vi "RGBtoLab.vi"() -> ()   [LabVIEW 8.6]
uses:
  <vilib>/vision/NI_Vision_Development_Module.lvlib
  <vilib>/vision/Image Controls.llb/IMAQ Image.ctl
panel:
  in  "File Path":path
  out "L out":T1
  out "a out":T1
  out "b out":T1
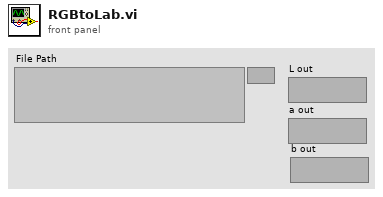
[diagram p1: front panel]
types:
  T1 = typedef "IMAQ Image.ctl" = refnum<image>
  T2 = typedef "Image Type" = u32
  T3 = cluster{"Red (or Hue) value":u8, "Green (or Sat) value":u8, "Blue (or Light or Val) value":u8}[][]
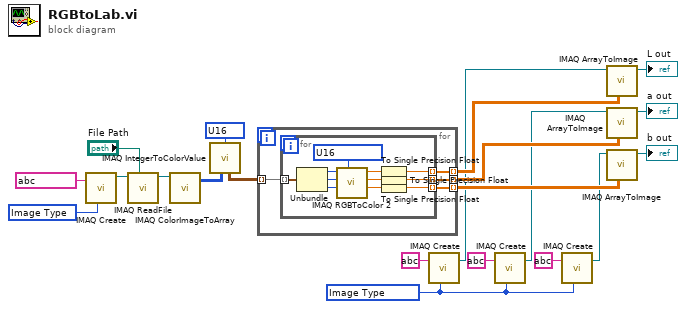
[diagram p0: block diagram]
diagram:
  w15 = T2 ? items=["Grayscale (U8)", "Grayscale (I16)", "Grayscale (SGL)", "Complex (CSG)", "RGB (U32)", "HSL (U32)", "RGB (U64)", "Grayscale (U16)"] ("Image Type")
  w3 = u16 ? items=["RGB", "HSL", "HSV", "HSI"] ("Color Mode")
  w1 = T2 ? items=["Grayscale (U8)", "Grayscale (I16)", "Grayscale (SGL)", "Complex (CSG)", "RGB (U32)", "HSL (U32)", "RGB (U64)", "Grayscale (U16)"] ("Image Type")
  n1 = call "IMAQ Create"("Image Name"=string ?, "Image Type"=w1) -> ("New Image"=w6:T1)  [unwired: 3 in, 1 out]
  n2 = call "IMAQ ReadFile"("File Path"="File Path", "Image"=w6) -> ("Image Out"=w7:T1)  [unwired: 5 in, 4 out]
  n3 = call "IMAQ ColorImageToArray"("Image"=w7) -> ("Image Pixels (U32)"=w2:u32[][])  [unwired: 2 in, 3 out]
  n4 = call "IMAQ IntegerToColorValue"("2D U32 array"=w2, "Color Mode"=w3) -> ("2D Color value array"=w4:T3)  [unwired: 3 in, 3 out]
  n5 = for {
    tunnel: w4 -> [w25] mode=indexing
    tunnel: [w24] -> w16 mode=indexing
    tunnel: [w23] -> w17 mode=indexing
    tunnel: [w22] -> w18 mode=indexing
    n6 = for {
      tunnel: w25 -> [w36] mode=indexing
      tunnel: [w32] -> w24 mode=indexing
      tunnel: [w28] -> w23 mode=indexing
      tunnel: [w27] -> w22 mode=indexing
      w26 = u16 ? items=["RGB", "HSL", "HSV", "HSI", "CIE L*a*b*", "CIE XYZ"] ("Color Mode")
      n7 = Unbundle(w36) -> ("Red (or Hue) value"=w35:u8, "Green (or Sat) value"=w34:u8, "Blue (or Light or Val) value"=w33:u8)
      n8 = call "IMAQ RGBToColor 2"("Color Mode"=w26, "Blue value"=w33, "Green value"=w34, "Red value"=w35) -> ("Blue or Luma or Val or Inten or Z or b*value"=w29:dbl, "Green or Sat or Y or a* value"=w30:dbl, "Red or Hue or X or L* value"=w31:dbl)  [unwired: 3 in, 2 out]
      n9 = To Single Precision Float(number=w31) -> (single precision float=w32:sgl)
      n10 = To Single Precision Float(number=w30) -> (single precision float=w28:sgl)
      n11 = To Single Precision Float(number=w29) -> (single precision float=w27:sgl)
    }
  }
  n12 = call "IMAQ Create"("Image Name"=string ?, "Image Type"=w15) -> ("New Image"=w14:T1)  [unwired: 3 in, 1 out]
  n13 = call "IMAQ Create"("Image Name"=string ?, "Image Type"=w15) -> ("New Image"=w13:T1)  [unwired: 3 in, 1 out]
  n14 = call "IMAQ Create"("Image Name"=string ?, "Image Type"=w15) -> ("New Image"=w12:T1)  [unwired: 3 in, 1 out]
  n15 = call "IMAQ ArrayToImage"("Image Pixels (Float)"=w16, "Image"=w14) -> ("Image Out"=→"L out":T1)  [unwired: 4 in, 5 out]
  n16 = call "IMAQ ArrayToImage"("Image Pixels (Float)"=w17, "Image"=w13) -> ("Image Out"=→"a out":T1)  [unwired: 4 in, 5 out]
  n17 = call "IMAQ ArrayToImage"("Image Pixels (Float)"=w18, "Image"=w12) -> ("Image Out"=→"b out":T1)  [unwired: 4 in, 5 out]
